vi "01.Wiener Filter - Color.vi"() -> (3 "dst image (reconstructed)":picture, 11 "src image (blurred)":picture)   [LabVIEW 2012]
doc: "This example showing the use case of Wiener Filter in imageprocessing. Wiener filter is a method of restoring image in the presence of blur (and noise) in the case when the blur kernel is known. In the given example I using Gaussian blur. This algorithm also can be used from restoring “motion blurred” images.\n\nA blurred or degraded image can be approximately described by equation Dst(x,y) = PSF * Src(x,y), where Src and Dst are source and result images and PSF is distortion operator called Point Spread Function. The Wiener filter can be understood better in the frequency domain. For deconvolution we will perform Fourier Transform of the blurred image, then perform convolution with inversed PSF function, and after inverse Fourier transform we will get the original image. When you know the exact PSF, the results of deblurring can be really effective."
uses:
  <vilib>/Analysis/2dsp.llb/2D Real FFT.vi
  <vilib>/Analysis/2dsp.llb/2D Inverse Real FFT.vi
  <vilib>/Analysis/NI_AALPro.lvlib
panel:
  in  "Sigma":dbl=3.0 min=1.0 max=3.0 step=0.1 format="%_3g"
  # "Color Wiener Filter Example"
  # "Wiener"
  # "Filter"
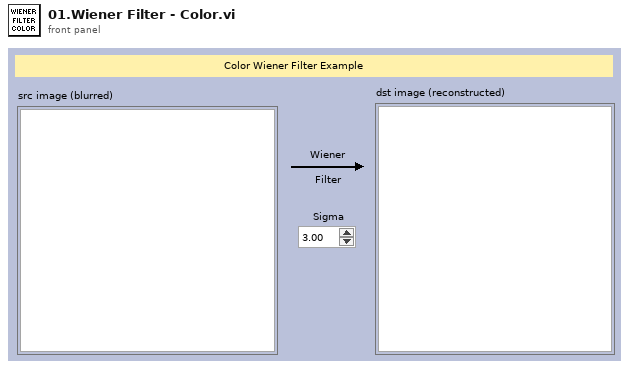
[diagram p1: front panel]
types:
  T1 = typedef "imagedata.ctl" = cluster{"image type":i32, "image depth":i32, "image":u8[], "mask":u8[], "colors":u32[], "Rectangle":cluster{"left":i16, "top":i16, "right":i16, "bottom":i16}}
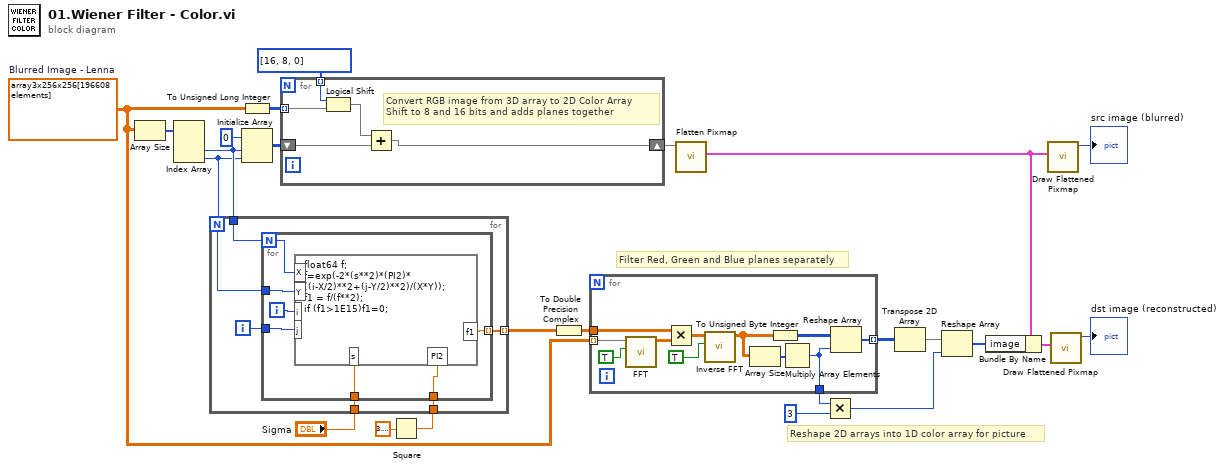
[diagram p0: block diagram]
diagram:
  w1 = dbl[][][] array3x256x256[196608 elements]  # Blurred Image - Lenna
  # "Filter Red, Green and Blue planes separately"
  # "Reshape 2D arrays into 1D color array for picture"
  n1 = Array Size(array=w1) -> (size(s)=w11:i32[])
  n2 = Index Array(array=w11) -> (element #2=w9:i32, element #3=w8:i32)  [unwired: 3 in, 1 out]
  n3 = To Unsigned Long Integer(number=w1) -> (unsigned 32bit integer=w17:u32[][][])
  n4 = Initialize Array(u32 0 ("dimension size"), w9, w8) -> (w15:u32[][])
  n5 = for {
    tunnel: w17 -> [w28] mode=indexing
    shift-right: [w29] -> w14
    shift-left: w15 -> [w27]
    tunnel: i32[] [16, 8, 0] ("unsharp image") -> [w25] mode=indexing
    # "Convert RGB image from 3D array to 2D Color Array\nShift to 8 and 16 bits and adds planes together"
    n6 = Logical Shift(y=w25, x=w28) -> (x << y=w26:u32[][])
    n7 = Add(x=w26, y=w27) -> (x+y=w29:u32[][])
  }
  n8 = Square(x=3.141592653589793) -> (x^2=w2:dbl)
  n9 = for {
    N: w8 -> [w34]
    tunnel: "Sigma" -> [w35]
    tunnel: [w32] -> w5 mode=indexing
    tunnel: w9 -> [w31]
    tunnel: w2 -> [w30]
    i -> [w33]
    n10 = for {
      N: w31 -> [w41]
      tunnel: w35 -> [w42]
      tunnel: w34 -> [w40]
      tunnel: w33 -> [w38]
      tunnel: [w37] -> w32 mode=indexing
      tunnel: w30 -> [w36]
      i -> [w39]
      # "PSF Function - Inverse Gauss"
      n11 = formula code="float64 f;\nf=exp(-2*(s**2)*(PI2)*\n((i-X/2)**2+(j-Y/2)**2)/(X*Y));\nf1 = f/(f**2);\nif (f1>1E15)f1=0;"("s"=w42, "X"=w41, "i"=w39, "j"=w38, "PI2"=w36, "Y"=w40) -> ("f1"=w37:dbl)
    }
  }
  n12 = To Double Precision Complex(1:w5) -> (0:w4:cdb[][])
  n13 = for {
    tunnel: [w49] -> w23 mode=indexing
    tunnel: [w48] -> w19
    tunnel: w1 -> [w47] mode=indexing
    tunnel: w4 -> [w45]
    n14 = call-poly <vilib>:"FFT.vi"("shift?"=TRUE, "X"=w47) -> ("FFT {X}"=w43:cdb[][])  [unwired: 8 in, 1 out]
    n15 = Multiply(x=w45, y=w43) -> (x*y=w46:cdb[][])
    n16 = call-poly <vilib>:"Inverse FFT.vi"("shift?"=TRUE, "FFT {X}"=w46) -> ("X"=w50:dbl[][])  [unwired: 8 in, 1 out]
    n17 = Array Size(array=w50) -> (size(s)=w51:i32[])
    n18 = To Unsigned Byte Integer(number=w50) -> (unsigned 8bit integer=w44:u8[][])
    n19 = Multiply Array Elements(1:w51) -> (0:w48:i32)
    n20 = Reshape Array(w44, w48) -> (w49:u8[])
  }
  n21 = call <vilib>:"Flatten Pixmap.vi"("24-bit pixmap"=w14) -> ("image data"=w13:T1)  [unwired: 10 in]
  n22 = Multiply(x=w19, y=3 ("x")) -> (x*y=w22:i32)
  n23 = Transpose 2D Array(2D array=w23) -> (transposed array=w20:u8[][])
  n24 = Reshape Array(w20, w22) -> (w21:u8[])
  n25 = Bundle By Name(cluster=w13, "image"=w21) -> (w24:T1)
  n26 = call <vilib>:"Draw Flattened Pixmap.vi"("image data"=w13) -> ("new picture"=→"src image (blurred)":picture)  [unwired: 8 in]
  n27 = call <vilib>:"Draw Flattened Pixmap.vi"("image data"=w24) -> ("new picture"=→"dst image (reconstructed)":picture)  [unwired: 8 in]
